vi "niRFUtil MT UTIL Apply Frequency Offset.vi"(0 "Signal In":T1 format="%.2f", 5 "Rate (S/s)":dbl format="%.2f", 7 "Freq Offset (Hz)":dbl format="%.2f", 9 "Initial Phase (deg)":dbl format="%.2f", 11 "error in (no error)":errorcluster, 13 "Reset? (T)":bool=TRUE) -> (4 "Signal Out":T1 format="%.2f", 15 "error out":errorcluster)   [LabVIEW 2015, in "niRFUtil.lvlib"]
doc: "Applies the given frequency offset to the signal. The function can be used as an impairment or as a corrector by simply entering the proper frequency offset. The incoming signal can be either samples or symbols: the \"Rate, pts/sec\" is simply a generic rate input to indicate the distance between points. Typically, though, this is run against sampled data, so that \"Rate\" is equivalent to \"Samples/Sec\".\n\nThe VI is memory-aware in that it can be called to \"continue\" to appy the frequency offset where it last left off by setting \"Reset\" to False.\n\nThis function is used by the IQ Impairments and the demodulators."
uses:
  niRFUtil.lvlib
  Includes/niRFUtil INC Complex Array.ctl
  niRFUtil MT UTIL Apply Frequency Offset (Complex SGL).vi
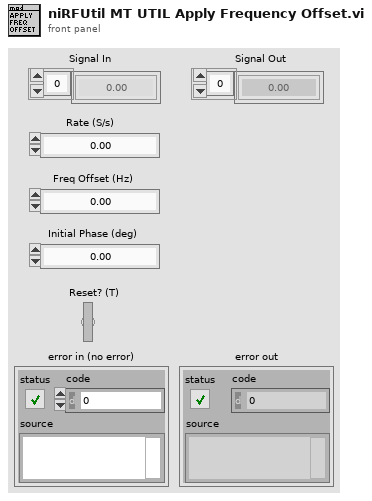
[diagram p1: front panel]
types:
  T1 = typedef "niRFUtil.lvlib/niRFUtil INC Complex Array.ctl" = csg[]
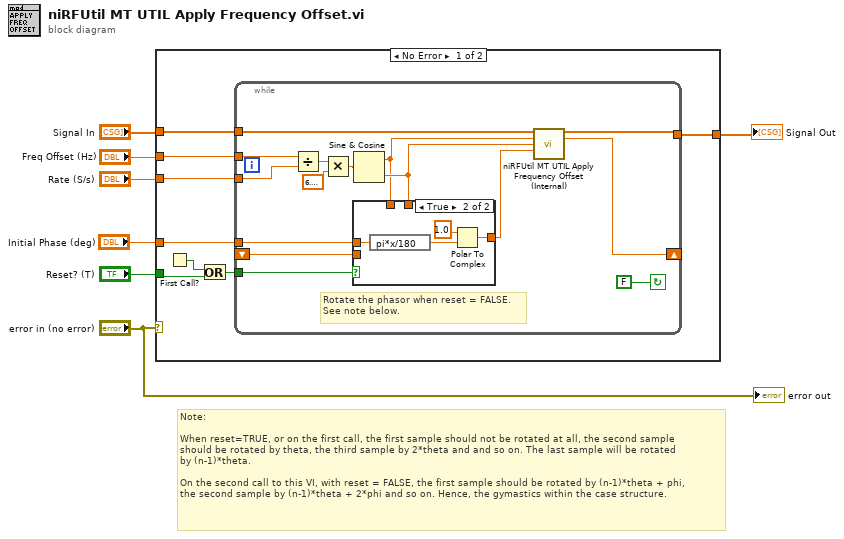
[diagram p0: block diagram]
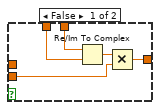
[diagram p2: hidden frame]
diagram:
  # "Note:\n\nWhen reset=TRUE, or on the first call, the first sample should not be rotated at all, the second sample \nshould be rotated by theta, the third sample by 2*theta and and so on. The last sample will be rotated\nby (n-1)*theta. \n\nOn the second call to this VI, with reset = FALSE, the first sample should be rotated by (n-1)*theta + phi,\nthe second sample by (n-1)*theta + 2*phi and so on. Hence, the gymastics within the case structure."
  n1 = case shown="No Error" "error in (no error)" {
    tunnel: "Signal In" -> [w15 _]
    tunnel: "Freq Offset (Hz)" -> [w14 _]
    tunnel: "Rate (S/s)" -> [w13 _]
    tunnel: "Reset? (T)" -> [w11 _]
    tunnel: [w9 _] -> w2
    tunnel: "Initial Phase (deg)" -> [w8 _]
    frame No Error {
      n2 = First Call?() -> (First Call?: T/F=w12:bool)
      n3 = Or(x=w12, y=w11) -> (x .or. y?=w10:bool)
      n4 = while {
        tunnel: w15 -> [w22]
        tunnel: w14 -> [w24]
        tunnel: w13 -> [w23]
        tunnel: w10 -> [w29]
        shift-right: [w20] -> _
        shift-left: _ -> [w28]
        tunnel: [w21] -> w9
        tunnel: w8 -> [w16]
        stop <- FALSE continue-if-true
        # "Rotate the phasor when reset = FALSE.\nSee note below."
        n5 = Divide(x=w24, y=w23) -> (x/y=w26:dbl)
        n6 = Multiply(x=w26, y=6.283185307179586) -> (x*y=w27:dbl)
        n7 = Sine & Cosine(0:w27) -> (1:w17:dbl, 2:w18:dbl)
        n8 = case shown="True" w29 {
          tunnel: w28 -> [w31 _]
          tunnel: [w32 w39] -> w19
          tunnel: w18 -> [w35 _]
          tunnel: w17 -> [w34 _]
          tunnel: w16 -> [_ w37]
          frame False {
            n9 = Re/Im To Complex(1:w34, 2:w35) -> (0:w33:cdb)
            n10 = Multiply(x=w33, y=w31) -> (x*y=w32:cdb)
          }
          frame True {
            n11 = expression code="pi*x/180"(w37) -> (w36:dbl)
            n12 = Polar To Complex(1:w36, 2:1.0 ("r")) -> (0:w39:cdb)
          }
        }
        n13 = call-poly "niRFUtil MT UTIL Apply Frequency Offset (Internal).vi"("Signal In"=w22, "sine"=w17, "cosine"=w18, "real (phasor) in"=w19) -> ("Signal Out"=w21:T1, "phasor out"=w20:cdb)  [unwired: 10 in]
      }
    }
    frame Error {
    }
  }
  "Signal Out" <- w2
  "error out" <- "error in (no error)"
